vi "create marker.vi"(2 "Location":string, 3 "Label {A-Z, 0-9}":string, 4 "Color":u32(colorbox)=36351, 5 "Size":string(combo)="mid", 6 "Icon URL":string) -> (0 "Marker String":string)   [LabVIEW 2012]
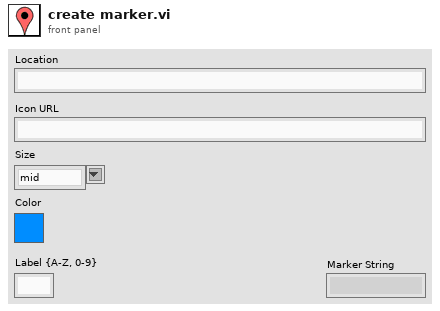
[diagram p1: front panel]
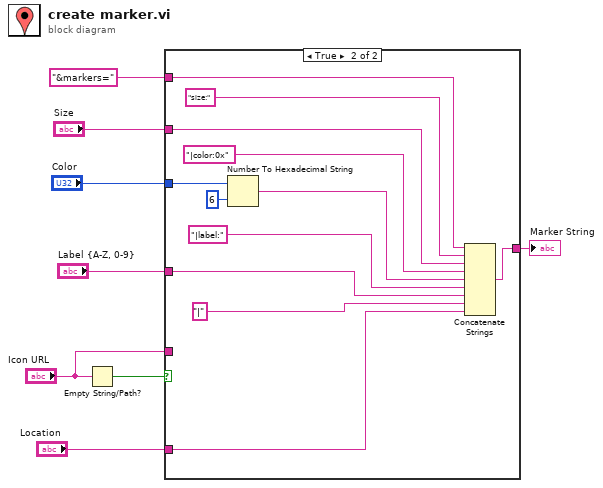
[diagram p0: block diagram]
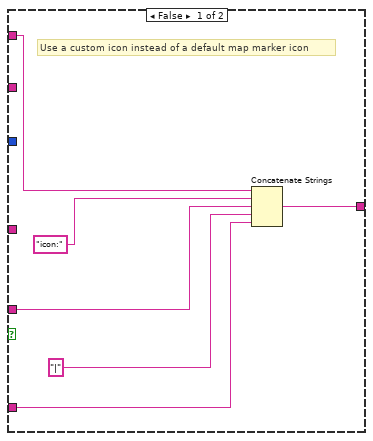
[diagram p2: hidden frame]
diagram:
  n1 = Empty String/Path?(string/path="Icon URL") -> (empty?=w8:bool)
  n2 = case shown="True" w8 {
    tunnel: "&markers=" -> [w14 w26]
    tunnel: "Icon URL" -> [w12 _]
    tunnel: "Location" -> [w10 w16]
    tunnel: [w9 w20] -> w4
    tunnel: "Size" -> [_ w24]
    tunnel: "Color" -> [_ w22]
    tunnel: "Label {A-Z, 0-9}" -> [_ w18]
    frame False {
      # "Use a custom icon instead of a default map marker icon"
      n3 = Concatenate Strings(w14, "icon:", w12, "|", w10) -> (w9:string)
    }
    frame True {
      n4 = Number To Hexadecimal String(1:i16 6 ("width (-)"), 2:w22) -> (0:w21:string)
      n5 = Concatenate Strings(w26, "size:", w24, "|color:0x", w21, "|label:", w18, "|", w16) -> (w20:string)
    }
  }
  "Marker String" <- w4
